vi "WriteConfiguration_Control.vi"(7 "PythonConverter_GUI in":refnum<class "PythonConverter_GUI.lvclass">, 8 "error in":errorcluster, 11 "Control in":refnum<class "Control.lvclass">) -> (0 "error out":errorcluster, 3 "Control out":refnum<class "Control.lvclass">, 5 "PythonConverter_GUI out":refnum<class "PythonConverter_GUI.lvclass">)   [LabVIEW 2014, in "Raspberry Pi Compatible Compiler for LabVIEW.lvlib" / "PythonConverter_GUI.lvclass"]
uses:
  PythonConverter_GUI.lvclass
  VI Interpreter/Classes/Control/Control.lvclass
  PythonConverter_GUI.lvclass/PythonConverter_GUI.ctl
  PythonConfiguration/PythonConfiguration.lvclass/PythonConfiguration.ctl
  VI Interpreter/Classes/GObject/GObject.lvclass/GObject.ctl
  VI Interpreter/Classes/Control/Control.lvclass/Control.ctl
  PythonConfiguration/PythonConfiguration.lvclass
  VI Interpreter/Classes/GObject/GObject.lvclass
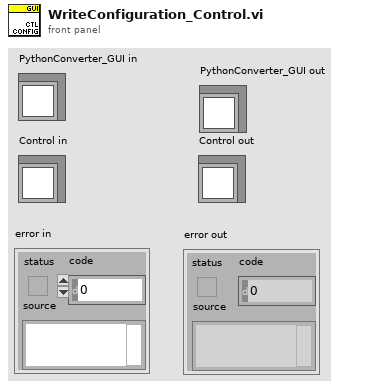
[diagram p1: front panel]
types:
  T1 = typedef "LVBoundsTypeDef.ctl" = cluster{"Width":u32, "Height":u32}
  T2 = typedef "Raspberry Pi Compatible Compiler for LabVIEW.lvlib/PythonConfiguration.lvclass/ItemTD.ctl" = cluster{"Key":string, "Value":string}
  T3 = typedef "LVPositionTypeDef.ctl" = cluster{"Left":i32, "Top":i32}
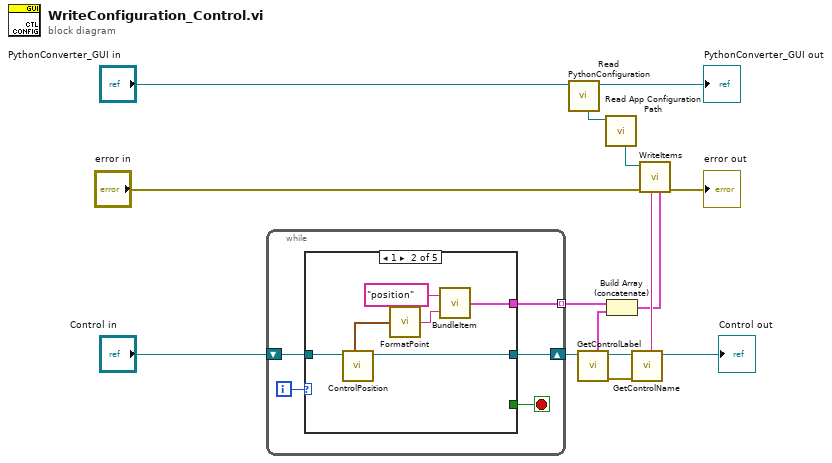
[diagram p0: block diagram]
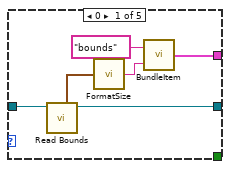
[diagram p2: hidden frame]
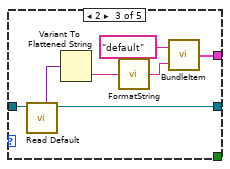
[diagram p3: hidden frame]
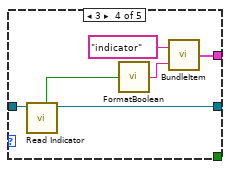
[diagram p4: hidden frame]
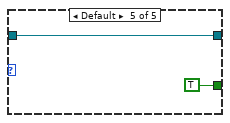
[diagram p5: hidden frame]
diagram:
  n1 = while {
    shift-right: [w18] -> w8
    shift-left: "Control in" -> [w19]
    tunnel: [w17] -> w15 mode=indexing
    i -> [w20]
    stop <- w16 stop-if-true
    n2 = case shown="1" w20 {
      tunnel: w19 -> [w24 w30 w36 w44 w47]
      tunnel: [w23 w29 w35 w43 w47] -> w18
      tunnel: [w22 w28 w34 w42 _] -> w17
      tunnel: [_ _ _ _ TRUE] -> w16
      frame 0 {
        n3 = call "Read Bounds.vi"("GObject in"=w24) -> ("GObject out"=w23:refnum<class "Control.lvclass">, "Bounds"=w21:T1)  [unwired: 7 in]
        n4 = call "FormatSize.vi"("size"=w21) -> ("value"=w25:string)
        n5 = call "BundleItem.vi"("Value"=w25, "Key"="bounds") -> ("Item"=w22:T2)
      }
      frame 1 {
        n6 = call-dynamic "ControlPosition.vi"("Control in"=w30) -> ("Control out"=w29:refnum<class "Control.lvclass">, "Position"=w27:T3)  [unwired: 6 in, 1 out]
        n7 = call "FormatPoint.vi"("point"=w27) -> ("value"=w31:string)
        n8 = call "BundleItem.vi"("Value"=w31, "Key"="position") -> ("Item"=w28:T2)
      }
      frame 2 {
        n9 = call "Read Default.vi"("Control in"=w36) -> ("Control out"=w35:refnum<class "Control.lvclass">, "Default"=w37:variant)  [unwired: 7 in]
        n10 = Variant To Flattened String(Variant=w37) -> (data string=w33:string)  [unwired: 1 out]
        n11 = call "FormatString.vi"("String"=w33) -> ("value"=w38:string)  [unwired: 1 in]
        n12 = call "BundleItem.vi"("Value"=w38, "Key"="default") -> ("Item"=w34:T2)
      }
      frame 3 {
        n13 = call "Read Indicator.vi"("Control in"=w44) -> ("Control out"=w43:refnum<class "Control.lvclass">, "Indicator"=w40:bool)  [unwired: 7 in]
        n14 = call "FormatBoolean.vi"("boolean"=w40) -> ("value"=w41:string)
        n15 = call "BundleItem.vi"("Value"=w41, "Key"="indicator") -> ("Item"=w42:T2)
      }
      frame Default {
      }
    }
  }
  n16 = call "Read PythonConfiguration.vi"("PythonConverter_GUI in"="PythonConverter_GUI in") -> ("PythonConverter_GUI out"=→"PythonConverter_GUI out":refnum<class "PythonConverter_GUI.lvclass">, "PythonConfiguration"=w12:refnum<class "PythonConfiguration.lvclass">)  [unwired: 7 in]
  n17 = call "GetControlLabel.vi"("Control in"=w8) -> ("error out"=w6:errorcluster, "Control out"=w7:refnum<class "Control.lvclass">, "Items"=w4:T2[])  [unwired: 6 in]
  n18 = call "Read App Configuration Path.vi"("PythonConfiguration in"=w12) -> ("App Configuration Path"=w11:path)  [unwired: 7 in, 1 out]
  n19 = Build Array (concatenate)(w15, w4) -> (w5:T2[])
  n20 = call "GetControlName.vi"("error in"=w6, "Control in"=w7) -> ("Control out"=→"Control out":refnum<class "Control.lvclass">, "name"=w14:string)  [unwired: 5 in, 1 out]
  n21 = call "WriteItems.vi"("Items"=w5, "section"=w14, "error in"="error in", "Path"=w11) -> ("error out"=→"error out":errorcluster)  [unwired: 5 in]
